vi "UHR-Fleezers Control (host) - 10.8.vi"() -> ()   [LabVIEW 2013] (continued)
          tunnel: [w3020] -> w2914 mode=indexing
          workers-P: _ -> [_]
          n1651 = Reverse 1D Array(array=w3021) -> (reversed array=w3020:dbl[])
        }
        n1652 = for {
          tunnel: w2989 -> [w3029] mode=indexing
          tunnel: [w3028] -> w2988 mode=indexing
          workers-P: _ -> [_]
          n1653 = Reverse 1D Array(array=w3029) -> (reversed array=w3028:dbl[])
        }
        n1654 = for {
          tunnel: w2978 -> [w3025] mode=indexing
          tunnel: [w3024] -> w2977 mode=indexing
          workers-P: _ -> [_]
          n1655 = Reverse 1D Array(array=w3025) -> (reversed array=w3024:dbl[])
        }
        n1656 = Index Array(array=w2990, index (row)=0) -> (element=→"Waveform Graph":dbl[])  [unwired: 1 in]
        n1657 = Add(x=w2984, y=w2983) -> (x+y=w2982:dbl[][])
        n1658 = Add(x=w2970, y=w2969) -> (x+y=w2968:dbl[][])
        n1659 = Add(x=w2914, y=w2913) -> (x+y=w2898:dbl[][])
        n1660 = Add(x=w2988, y=w2987) -> (x+y=w2962:dbl[][])
        n1661 = Add(x=w2977, y=w2976) -> (x+y=w2975:dbl[][])
        n1662 = Divide(x=w2968, y=2) -> (x/y=w2966:dbl[][])
        n1663 = Divide(x=w2982, y=2) -> (x/y=w2927:dbl[][])
        n1664 = Divide(x=w2975, y=2) -> (x/y=w2929:dbl[][])
        n1665 = To Single Precision Float(number=w2962) -> (single precision float=w2961:sgl[][])
        n1666 = Transpose 2D Array(2D array=w2966) -> (transposed array=→"Data map":dbl[][])
        n1667 = To Single Precision Float(number=w2898) -> (single precision float=w2902:sgl[][])
        n1668 = To Single Precision Float(number=w2927) -> (single precision float=w2933:sgl[][])
        n1669 = To Single Precision Float(number=w2929) -> (single precision float=w2930:sgl[][])
        n1670 = call "IMAQ ArrayToImage"("Image Pixels (Float)"=w2961, "Image"=w2895) -> ("Image Out"=w2964:T2)  [unwired: 8 in, 1 out]
        n1671 = call "IMAQ ArrayToImage"("Image Pixels (Float)"=w2902, "Image"=w2894) -> ("Image Out"=w2904:T2)  [unwired: 8 in, 1 out]
        n1672 = call "IMAQ ArrayToImage"("Image Pixels (Float)"=w2933, "Image"=w2893) -> ("Image Out"=w2935:T2)  [unwired: 8 in, 1 out]
        n1673 = call "IMAQ ArrayToImage"("Image Pixels (Float)"=w2930, "Image"=w2892) -> ("Image Out"=w2932:T2)  [unwired: 8 in, 1 out]
        n1674 = call "IMAQ Symmetry"("Type of Symmetry"=w2963, "Image Src"=w2964) -> ("Image Dst Out"=w2959:T2)  [unwired: 3 in, 1 out]
        n1675 = call "IMAQ Symmetry"("Type of Symmetry"=w2903, "Image Src"=w2904) -> ("Image Dst Out"=w2900:T2)  [unwired: 3 in, 1 out]
        n1676 = call "IMAQ Symmetry"("Type of Symmetry"=w2934, "Image Src"=w2935) -> ("Image Dst Out"=→"Detection Laser X":T2)  [unwired: 3 in, 1 out]
        n1677 = call "IMAQ Symmetry"("Type of Symmetry"=w2931, "Image Src"=w2932) -> ("Image Dst Out"=→"Detection Laser Y":T2)  [unwired: 3 in, 1 out]
        n1678 = call "IMAQ Set Simple Calibration"("Calibration Axis Info"=T39 {"Origin Pixel"={"X"=0.0, "Y"=0.0}, "Angle Relative to Horizontal (deg)"=0.0, "Axis Reference"=0}, "Grid Descriptor"=T40 {"X Step"=0.3, "Y Step"=0.3, "Unit"=enum."Undefined"}, "Image"=w2959) -> ("Calibrated Image"=→"APD 1":T2)  [unwired: 7 in, 1 out]
        n1679 = call "IMAQ Set Simple Calibration"("Calibration Axis Info"=T39 {"Origin Pixel"={"X"=0.0, "Y"=0.0}, "Angle Relative to Horizontal (deg)"=0.0, "Axis Reference"=0}, "Grid Descriptor"=T40 {"X Step"=0.3, "Y Step"=0.3, "Unit"=enum."Undefined"}, "Image"=w2900) -> ("Calibrated Image"=→"APD 2":T2)  [unwired: 7 in, 1 out]
      }
    }
    n1680 = Subtract(x=w1995, y="APD 2 Offset") -> (x-y=w1992:waveform(dbl))
    n1681 = Subtract(x=w1997, y="APD 1 Offset") -> (x-y=w1993:waveform(dbl))
    n1682 = Index Array(array=w2012, index=3) -> (element=w2081:waveform(dbl))
    n1683 = Index Array(array=w2012, index=6) -> (element=w2078:waveform(dbl))
    n1684 = Build Array(w1993, w1992) -> (→"APD Chart":waveform(dbl)[])
    n1685 = Array Size(array=w2070) -> (size(s)=w2125:i32)
    n1686 = call <vilib>:"Std Deviation and Variance.vi"("X"=w2005) -> ("standard deviation"=w2004:dbl)  [unwired: 1 in, 2 out]
    n1687 = Add Array Elements(numeric array=w2005) -> (sum=w2007:u32)
    n1688 = Add Array Elements(numeric array=w2070) -> (sum=w2135:u32)
    n1689 = call <vilib>:"Std Deviation and Variance.vi"("X"=w2070) -> ("standard deviation"=w2069:dbl)  [unwired: 1 in, 2 out]
    n1690 = Divide(x="T1 offset_x (mV)", y=1000.0) -> (x/y=w2082:dbl)
    n1691 = Divide(x=w2004, y=w2003) -> (x/y=w2000:dbl)
    "Rate sigma (Hz) 2" <- w2000
    n1692 = Multiply(x=w2003, y=w2125) -> (x*y=w2006:dbl)
    "Int. Time (s)" <- w2006
    n1693 = Divide(x=w2007, y=w2006) -> (x/y=w2001:dbl)
    "APD 2 Rate (Hz)" <- w2001
    n1694 = Divide(x=w2135, y=w2006) -> (x/y=w2067:dbl)
    "APD 1 Rate (Hz)" <- w2067
    n1695 = Divide(x=w2069, y=w2003) -> (x/y=w2068:dbl)
    "Rate sigma (Hz)" <- w2068
    n1696 = Divide(x=w2000, y=w2001) -> (x/y=→"Sigma/Mean 2":dbl)
    n1697 = Divide(x=w2068, y=w2067) -> (x/y=→"Sigma/Mean":dbl)
    n1698 = Divide(x="T2 offset_x (mV)", y=1000.0) -> (x/y=w2080:dbl)
    n1699 = case shown="1" "Calibration" {
      tunnel: "T1 alpha_x (nm/V)" -> [_ w2858 w2879]
      tunnel: "T1 kappa_x (pN/nm)" -> [_ _ w2869]
      tunnel: "T2 alpha_x (nm/V)" -> [_ w2857 w2877]
      tunnel: "T2 kappa_x (pN/nm)" -> [_ _ w2870]
      tunnel: w2081 -> [w2840 w2855 w2875]
      tunnel: w2078 -> [w2839 w2853 w2873]
      tunnel: [w2840 w2852 w2872] -> w2111
      tunnel: [w2839 w2851 w2871] -> w2110
      tunnel: ["T1 X (V)" ("Label.Text") "T1 X (nm)" ("Label.Text") "T1 X (pN)" ("Label.Text")] -> w2099
      tunnel: ["T2 X (V)" ("Label.Text") "T2 X (nm)" ("Label.Text") "T2 X (pN)" ("Label.Text")] -> w2098
      tunnel: ["Position (V)" ("Label.Text") "Position (nm)" ("Label.Text") "Force (pN)" ("Label.Text")] -> w2100
      tunnel: w2080 -> [_ w2843 w2862]
      tunnel: w2082 -> [_ w2846 w2864]
      tunnel: ["Mean (V)" ("Label.Text") "Mean (nm)" ("Label.Text") "Mean (pN)" ("Label.Text")] -> w2095
      tunnel: ["Difference (V)" ("Label.Text") "Difference (nm)" ("Label.Text") "Difference (pN)" ("Label.Text")] -> w2020
      frame 0, Default {
      }
      frame 1 {
        # "position"
        n1700 = Unbundle By Name(w2855) -> ("Y"=w2859:dbl[])
        n1701 = Unbundle By Name(w2853) -> ("Y"=w2844:dbl[])
        n1702 = Subtract(x=w2859, y=w2846) -> (x-y=w2847:dbl[])
        n1703 = Subtract(x=w2844, y=w2843) -> (x-y=w2845:dbl[])
        n1704 = Multiply(x=w2845, y=w2857) -> (x*y=w2854:dbl[])
        n1705 = Multiply(x=w2858, y=w2847) -> (x*y=w2856:dbl[])
        n1706 = Bundle By Name(cluster=w2853, "Y"=w2854) -> (w2851:waveform(dbl))
        n1707 = Bundle By Name(cluster=w2855, "Y"=w2856) -> (w2852:waveform(dbl))
      }
      frame 2 {
        # "force"
        n1708 = Unbundle By Name(w2875) -> ("Y"=w2880:dbl[])
        n1709 = Unbundle By Name(w2873) -> ("Y"=w2878:dbl[])
        n1710 = Subtract(x=w2878, y=w2862) -> (x-y=w2863:dbl[])
        n1711 = Subtract(x=w2880, y=w2864) -> (x-y=w2865:dbl[])
        n1712 = Compound Arithmetic op=MULTIPLY(w2863, w2877, w2870) -> (w2874:dbl[])
        n1713 = Compound Arithmetic op=MULTIPLY(w2869, w2879, w2865) -> (w2876:dbl[])
        n1714 = Bundle By Name(cluster=w2873, "Y"=w2874) -> (w2871:waveform(dbl))
        n1715 = Bundle By Name(cluster=w2875, "Y"=w2876) -> (w2872:waveform(dbl))
      }
    }
    n1716 = feedback-in #17("Calibration") -> ()
    n1717 = feedback #17(u16 1 ("Calibration")) -> (w2102:u16)
    n1718 = Not Equal?(x=w2102, y="Calibration") -> (x != y?=w2058:bool)
    n1719 = Unbundle By Name(w2081) -> ("Y"=w2084:dbl[])
    n1720 = Unbundle By Name(w2078) -> ("Y"=w2087:dbl[])
    n1721 = Subtract(x=w2084, y=w2082) -> (x-y=w2085:dbl[])
    n1722 = Subtract(x=w2087, y=w2080) -> (x-y=w2086:dbl[])
    n1723 = disable-structure shown="Enabled" {
      disable-tunnel: [-1.0 ("y") 1.0] -> w2088
      frame Disabled {
      }
      frame Enabled {
      }
    }
    n1724 = Multiply(x=w2086, y="T2 alpha_x (nm/V)") -> (x*y=w2077:dbl[])
    n1725 = Multiply(x="T1 alpha_x (nm/V)", y=w2085) -> (x*y=w2076:dbl[])
    n1726 = Multiply(x=w2110, y=w2088) -> (x*y=w2089:waveform(dbl))
    n1727 = case shown="True" "Read Lateness and Rel Phase" {
      tunnel: w1912 -> [w2415 w2437]
      tunnel: w1911 -> [w2416 w2436]
      tunnel: [w2415 w2435] -> w2073
      tunnel: [w2416 w2434] -> w2072
      frame False {
      }
      frame True {
        n1728 = xnode "Read/Write Control"("FPGA VI Reference In"=w2437, "error in"=w2436) -> ("FPGA VI Reference Out"=w2435:T19, "error out"=w2434:errorcluster, "GI Relative phase"=→"GI relative phase":i16, "Relative phase"=→"Relative phase (AI1)":i16, "AI Late Counter"=→"Late Counter (AI1)":u16, "GI Late Counter"=→"GI Late Counter":u16, "MCL Late Counter"=→"MCL Late Counter":u16, "MCL Relative Phase"=→"Relative Phase (MCL)":i16, "APD Acq Relative Phase"=→"APD Acq Relative Phase":i16, "APD 1 Gate Relative Phase"=→"APD 1 Gate Relative Phase":i16, "APD 2 Gate Relative Phase"=→"APD 2 Gate Relative Phase":i16, "APD Acq Late Counter"=→"APD Acq Late Counter":u16, "APD 1 Gate Late Counter"=→"APD 1 Gate Late Counter":u16, "APD 2 Gate Late Counter"=→"APD 2 Gate Late Counter":u16, "Green FB Relative Phase"=→"Relative phase (Green FB)":i16, "GI Relative phase 2"=→"GI relative phase 2":i16, "GI Late Counter 2"=→"GI Late Counter 2":u16, "Trap Pos FIFO Timeout"=→"Trap Pos FIFO Timeout":u16, "Trap AI FIFO Timeout"=→"Trap AI FIFO Timeout":u16)
      }
    }
    n1729 = Subtract(x=w2077, y=w2076) -> (x-y=w2075:dbl[])
    n1730 = Unbundle By Name(w2110) -> ("Y"=w2045:dbl[])
    n1731 = Unbundle By Name(w2111) -> ("Y"=w2046:dbl[])
    n1732 = Build Array(w2111, w2089) -> (→"Force":waveform(dbl)[])
    n1733 = Subtract(x=w2075, y="Offset (nm)") -> (x-y=w2043:dbl[])
    n1734 = call-poly <vilib>:"Mean.vi"("X"=w2045) -> ("mean"=w2024:dbl)  [unwired: 1 out]
    "T2 X" <- w2024
    n1735 = Absolute Value(x=w2046) -> (abs(x)=w2047:dbl[])
    n1736 = Absolute Value(x=w2045) -> (abs(x)=w2048:dbl[])
    n1737 = call-poly <vilib>:"Mean.vi"("X"=w2046) -> ("mean"=w2025:dbl)  [unwired: 1 out]
    "T1 X" <- w2025
    n1738 = Add(x=w2047, y=w2048) -> (x+y=w2049:dbl[])
    n1739 = Bundle By Name(cluster=w2081, "Y"=w2043) -> (w2011:waveform(dbl))
    "Bead Separation" <- w2011
    n1740 = Divide(x=w2049, y=2.0) -> (x/y=→"Vec Mean of T1 T2":dbl[])
    n1741 = case shown="True" w2058 {
      tunnel: w2100 -> [_ w2833]
      tunnel: w2099 -> [_ w2832]
      tunnel: w2098 -> [_ w2831]
      tunnel: w2095 -> [_ w2830]
      tunnel: w2020 -> [_ w2829]
      frame False {
      }
      frame True {
        n1742 = property on="Force" class="WFChart (strict)"("YScale.NameLbl.Text"=w2833) -> ()  [unwired: 2 in, 2 out]
        n1743 = property on="T2 X" class="DigNum (strict)"("Caption.Text"=w2831) -> ()  [unwired: 2 in, 2 out]
        n1744 = property on="T1 X" class="DigNum (strict)"("Caption.Text"=w2832) -> ()  [unwired: 2 in, 2 out]
        n1745 = property on="Mean" class="DigNum (strict)"("Caption.Text"=w2830) -> ()  [unwired: 2 in, 2 out]
        n1746 = property on="Difference" class="DigNum (strict)"("Caption.Text"=w2829) -> ()  [unwired: 2 in, 2 out]
      }
    }
    n1747 = local read "Tether"() -> (w2052:bool)
    n1748 = Absolute Value(x=w2025) -> (abs(x)=w2022:dbl)
    n1749 = Absolute Value(x=w2024) -> (abs(x)=w2021:dbl)
    n1750 = Add(x=w2022, y=w2021) -> (x+y=w2097:dbl)
    n1751 = Subtract(x=w2022, y=w2021) -> (x-y=→"Difference":dbl)
    n1752 = feedback #18(w2043) -> (w2042:dbl[])
    n1753 = Divide(x=w2097, y=2.0) -> (x/y=w2051:dbl)
    "Mean" <- w2051
    n1754 = case shown="True" w2052 {
      tunnel: w2051 -> [_ w2374]
      frame False {
      }
      frame True {
        n1755 = Greater?(x="Lost Tether Alarm Threshold (pN)", y=w2374) -> (0:w2372:bool)
        n1756 = case shown="True" w2372 {
          frame False {
          }
          frame True {
            n1757 = flat-sequence {
              frame #0 {
                # "stop only if saving"
                n1758 = local read "Saving..."() -> (w2387:bool)
                n1759 = And(x=w2387, y="TA Cancel Save?") -> (x .and. y?=w2386:bool)
                n1760 = local write "Stop Saving"(w2386) -> ()
              }
              frame #1 {
                n1761 = case shown="True" "TA Green Off?" {
                  frame False {
                  }
                  frame True {
                    w2390 = FALSE ("Fl. Triggered...")
                    n1762 = local write "Fl. Triggered..."(w2390) -> ()
                    n1763 = property on="Green Laser ON/Interlacing" class="Bool (strict)"("Val(Sgnl)"=w2390) -> ()  [unwired: 2 in, 2 out]
                  }
                }
              }
            }
            n1764 = local read "Time tether formed"() -> (w2381:timestamp)
            n1765 = Get Date/Time In Seconds() -> (seconds since 1Jan1904=w2382:timestamp)
            n1766 = Subtract(x=w2382, y=w2381) -> (x-y=w2380:dbl)
            n1767 = Number To Decimal String(number=w2380) -> (decimal integer string=w2377:string)  [unwired: 1 out]
            n1768 = local read "Messages"() -> (w2384:string)
            n1769 = call <vilib>:"Beep.vi"() -> ()  [unwired: 3 in, 9 out]
            n1770 = Concatenate Strings("Lost tether (" ("Message to add"), w2377, " s)." ("string")) -> (w2379:string)
            n1771 = local write "Tether"(FALSE ("Tether")) -> ()
            n1772 = call "Update messages.vi"("Message to add"=w2379, "Old message string"=w2384) -> ("New message string"=w2383:string)
            n1773 = local write "Messages"(w2383) -> ()
            n1774 = property on="Trap Pos. FB ON" class="Bool (strict)"("Val(Sgnl)"=FALSE ("Value (Signaling)")) -> ()  [unwired: 2 in, 2 out]
          }
        }
      }
    }
    n1775 = Build Array (concatenate)(w2043, w2042) -> (w2041:dbl[])
    n1776 = Split 1D Array(array=w2041, index=w1923) -> (first subarray=w2037:dbl[])  [unwired: 1 out]
    n1777 = feedback-in #18(w2037) -> ()
    n1778 = call-poly <vilib>:"Mean.vi"("X"=w2037) -> ("mean"=w2036:dbl)  [unwired: 1 out]
    "Bead Mean (nm)" <- w2036
    n1779 = Subtract(x=w2037, y=w2036) -> (x-y=w2035:dbl[])
    n1780 = Square(x=w2035) -> (x^2=w2034:dbl[])
    n1781 = call-poly <vilib>:"Mean.vi"("X"=w2034) -> ("mean"=w2033:dbl)  [unwired: 1 out]
    n1782 = Square Root(x=w2033) -> (sqrt(x)=w2032:dbl)
    n1783 = Multiply(x=10.0, y=w2032) -> (x*y=→"RMS (Ang)":dbl)
    n1784 = xnode "Read/Write Control"("FPGA VI Reference In"=w2073, "error in"=w2072) -> ("FPGA VI Reference Out"=w2191:T19, "error out"=w2185:errorcluster, "AI2 Y Sum Set 1"=w2181:i16, "AI2 Y Sum Set 2"=w2180:i16, "AI1 X Set 1"=w1957:fxp<+/-,16,1>, "AI1 X Set 2"=w1956:fxp<+/-,16,1>, "Trap Pos FB Int Signal"=→"Trap Pos FB Int Signal":fxp<+/-,24,9>, "Trap Pos FB Int-Norm Signal"=→"Trap Pos FB Int-Norm Signal":fxp<+/-,16,1>, "Trap Pos FB Action"=w1950:i64, "Scanning"=→"AOD Scanning":bool, "Scan I"=→"AOD Scan I":u64, "Scanning MCL"=w2183:bool, "Scan I (MCL)"=→"MCL Scan I":u64, "Green FB Signals"=w2120:T44)  [unwired: 1 out]
    "MCL Scanning" <- w2183
    "Trap Pos FB Action" <- w1950
    n1785 = local read "AI2 (V)"() -> (w2182:cluster{"Set 1":dbl, "Set 2":dbl})
    n1786 = Bundle By Name(cluster=w2182, "Set 1"=w2181, "Set 2"=w2180) -> (w2178:cluster{"Set 1":dbl, "Set 2":dbl})
    n1787 = Divide(x=w1950, y=327.67) -> (x/y=→"Action (%)":dbl)
    n1788 = local read "Trap X (AI1)"() -> (w1970:T10)
    n1789 = Divide(x=w2178, y=3276.7) -> (x/y=w2177:cluster{"Set 1":dbl, "Set 2":dbl})
    n1790 = local write "AI2 (V)"(w2177) -> ()
    n1791 = Bundle(cluster=w1970, "Trap 1"=w1957, "Trap 2"=w1956) -> (→"Trap X (AI1)":T10)
    n1792 = Divide(x=w2120, y=3276.7) -> (x/y=w2116:T51)
    n1793 = Unbundle By Name(w2116) -> ("Green FB Ch 0"=w2119:dbl, "Green FB Ch 1"=w2118:dbl, "Green FB Ch 2"=w2117:dbl)
    n1794 = Divide(x=w2119, y=w2117) -> (x/y=w2115:dbl)
    n1795 = Divide(x=w2118, y=w2117) -> (x/y=w2114:dbl)
    n1796 = flat-sequence "To save data" {
      tunnel: [w4117] -> w2202
      tunnel: [w4118] -> w2201
      tunnel: w2151 -> [w4111]
      tunnel: w2039 -> [w4115]
      tunnel: ["Save Calibration"] -> w2174
      tunnel: w2171 -> [w4114]
      tunnel: [w4107] -> w2170
      tunnel: [w4104] -> w2169
      tunnel: [w4101] -> w2168
      tunnel: w2150 -> [w4103]
      tunnel: w2056 -> [w4097]
      tunnel: [w4097] -> w2055
      tunnel: ["Start Saving"] -> w2013
      tunnel: [w4091] -> w1939
      tunnel: [w4090] -> w1938
      tunnel: w2202 -> [w4352]
      tunnel: w2201 -> [w4351]
      tunnel: w1940 -> [w4350]
      tunnel: w2174 -> [w4349]
      tunnel: w2170 -> [w4347]
      tunnel: w2169 -> [w4346]
      tunnel: w2168 -> [w4345]
      tunnel: w2026 -> [w4344]
      tunnel: w2065 -> [w4343]
      tunnel: w2055 -> [w4342]
      tunnel: w2013 -> [w4341]
      tunnel: w2011 -> [w4340]
      tunnel: w1987 -> [w4339]
      tunnel: w1939 -> [w4338]
      tunnel: w1938 -> [w4337]
      tunnel: w1937 -> [w4336]
      frame #0 {
        n1797 = Or(x="Save N Sets", y="Start Saving") -> (x .or. y?=w4098:bool)
        n1798 = To Double Precision Float(number=w4114) -> (double precision float=w4108:dbl)
        n1799 = Build Array(w4098, "Save Calibration", w4111, w4103) -> (w4113:bool[])
        n1800 = Compound Arithmetic op=OR("Save Calibration", w4111, w4098, w4103) -> (w4116:bool)
        n1801 = Boolean Array To Number(Boolean array=w4113) -> (number=w4110:u32)
        n1802 = feedback #19(FALSE ("Save APD Data\nwith Trap Data")) -> (w4092:bool)
        n1803 = feedback #20(refnum<k0> refnum) -> (w4119:refnum<file>)
        n1804 = feedback #21(refnum<k0> refnum) -> (w4094:refnum<file>)
        n1805 = feedback #22(FALSE ("Save APD Data\nwith Trap Data")) -> (w4102:bool)
        n1806 = feedback #23(refnum<k0> refnum) -> (w4105:refnum<file>)
        n1807 = feedback #24(0) -> (w4121:i32)
        n1808 = feedback #25() -> (w4109:u32)  [unwired: 1 out]
        n1809 = case shown="True" w4116 {
          tunnel: [w4128 1] -> w4117
          tunnel: w4121 -> [w4130 _]
          tunnel: [w4129 w4148] -> w4118
          tunnel: w4119 -> [w4129 _]
          tunnel: w4115 -> [_ w4168]
          tunnel: w4108 -> [_ w4166]
          tunnel: w4110 -> [_ w4169]
          tunnel: [w4127 w4147] -> w4107
          tunnel: w4109 -> [w4127 _]
          tunnel: [w4126 w4145] -> w4104
          tunnel: w4105 -> [w4126 _]
          tunnel: [w4125 w4144] -> w4101
          tunnel: w4102 -> [w4125 _]
          tunnel: "Start Saving" -> [_ w4142]
          tunnel: w4097 -> [_ w4141]
          tunnel: [w4124 w4132] -> w4090
          tunnel: w4094 -> [w4124 _]
          tunnel: [w4123 w4131] -> w4091
          tunnel: w4092 -> [w4123 _]
          frame False {
            n1810 = Increment(x=w4130) -> (x+1=w4128:i32)
          }
          frame True {
            w4138 = FALSE ("Start Saving")
            w4143 = 9.0  # File Version
            w4151 = FALSE ("prepend array or string size? (T)")
            w4149 = T31."big-endian, network order" ("byte order (0:big-endian, network order)")
            # "write file headers"
            n1811 = local read "BD 1 Frequency 1 (MHz)"() -> (w4165:dbl)
            n1812 = local read "BD 2 Frequency 1 (MHz)"() -> (w4164:dbl)
            n1813 = local read "BD 1 Frequency 2 (MHz)"() -> (w4163:dbl)
            n1814 = local read "BD 2 Frequency 2 (MHz)"() -> (w4162:dbl)
            n1815 = local read "BD 1 Frequency 3 (MHz)"() -> (w4161:dbl)
            n1816 = local read "BD 2 Frequency 3 (MHz)"() -> (w4160:dbl)
            n1817 = Array Size(array=w4141) -> (size(s)=w4140:i32)
            n1818 = To Double Precision Float(number=w4140) -> (double precision float=w4139:dbl)
            n1819 = local write "Save Calibration"(w4138) -> ()
            n1820 = local write "Start Saving"(w4138) -> ()
            n1821 = Build Array("Save APD Data\nwith Trap Data", "Save Trap Pos. Data") -> (w4135:bool[])
            n1822 = Boolean Array To Number(Boolean array=w4135) -> (number=w4134:u32)
            n1823 = Build Array(w4165, w4164, w4163, w4162, w4161, w4160) -> (w4159:dbl[])
            n1824 = case shown="4" w4169 {
              tunnel: w4168 -> [w4240 w4260 w4276 w4314]
              tunnel: w4139 -> [w4245 w4267 w4296 w4333]
              tunnel: w4166 -> [w4244 w4266 w4295 w4332]
              tunnel: [w4241 w4262 w4287 w4324] -> w4157
              tunnel: [w4232 "Cal sets to save" w4277 w4315] -> w4147
              tunnel: w4159 -> [w4242 w4263 w4289 w4326]
              tunnel: "Save APD Data\nwith Trap Data" -> [w4239 _ w4273 w4312]
              tunnel: [w4239 w4254 w4273 w4312] -> w4144
              tunnel: w4143 -> [w4235 w4255 w4271 w4310]
              tunnel: w4142 -> [w4234 _ _ _]
              tunnel: [w4225 w4254 w4270 w4300] -> w4131
              tunnel: "Save Trap Pos. Data" -> [w4225 _ w4270 w4300]
              tunnel: w4134 -> [w4224 _ w4269 w4299]
              frame 1, Default {
                # "timeseries"
                n1825 = case shown="True" "Profile" {
                  tunnel: [w4248 w4251] -> w4229
                  tunnel: [w4248 w4250] -> w4228
                  tunnel: [w4248 w4249] -> w4227
                  tunnel: [w4248 w4253] -> w4226
                  frame False {
                    w4248 = 0.0 ("f")
                  }
                  frame True {
                    n1826 = local read "Current Position"() -> (w4252:dbl[])
                    n1827 = local read "Y change (mm)"() -> (w4253:dbl)
                    n1828 = call "subVI_explode3array.vi"("Array"=w4252) -> ("x"=w4251:dbl, "y"=w4250:dbl, "z"=w4249:dbl)  [unwired: 12 in]
                  }
                }
                n1829 = local read "Save ave N"() -> (w4247:dbl)
                n1830 = Multiply(x=w4247, y=w4240) -> (x*y=w4246:dbl)
                n1831 = To Double Precision Float(number=w4224) -> (double precision float=w4238:dbl)
                n1832 = Build Array(w4235, w4240, w4246, w4245, w4244, 0.0 ("f")) -> (w4243:dbl[])
                n1833 = Build Array(w4238, w4229, w4228, w4227, w4226) -> (w4236:dbl[])
                n1834 = Select(t=u32 4000000000, s=w4234, f="N sets to save") -> (s? t:f=w4232:u32)
                n1835 = Build Array (concatenate)(w4243, w4242, w4236) -> (w4241:dbl[])
              }
              frame 2 {
                w4257 = 0.0 ("f")
                w4254 = FALSE ("Save APD Data\nwith Trap Data")
                # "calibration"
                n1836 = Boolean To (0,1)(Boolean=w4254) -> (0, 1=w4259:i16)
                n1837 = To Double Precision Float(number=w4259) -> (double precision float=w4258:dbl)
                n1838 = Build Array(w4258, w4257, w4257, w4257, w4257) -> (w4256:dbl[])
                n1839 = Build Array(w4255, w4260, w4260, w4267, w4266, 1.0 ("t")) -> (w4264:dbl[])
                n1840 = Build Array (concatenate)(w4264, w4263, w4256) -> (w4262:dbl[])
                "Calibrating Trap..." <- TRUE ("Calibrating...")
              }
              frame 4 {
                w4274 = 0.0 ("f")
                # "write file header for a trap \nraster scan"
                # "scan dir (x/y = 0/1)"
                # "cycles/step"
                # "n scans (f/b)"
                # "steps"
                # "freq. range"
                # "AOD raster scan"
                n1841 = local read "Number of F/B Scans (AOD)"() -> (w4281:u16)
                n1842 = local read "Cycles/step (AOD)"() -> (w4283:u64)
                n1843 = local read "Scan Range (MHz)"() -> (w4286:dbl)
                n1844 = local read "Scan steps (AOD)"() -> (w4285:u64)
                n1845 = local read "Scan BD"() -> (w4293:bool)
                n1846 = local read "Save ave N"() -> (w4298:dbl)
                n1847 = Boolean To (0,1)(Boolean=w4293) -> (0, 1=w4292:i16)
                n1848 = To Double Precision Float(number=w4281) -> (double precision float=w4280:dbl)
                n1849 = To Double Precision Float(number=w4285) -> (double precision float=w4284:dbl)
                n1850 = To Double Precision Float(number=w4283) -> (double precision float=w4282:dbl)
                n1851 = To Double Precision Float(number=w4292) -> (double precision float=w4291:dbl)
                n1852 = Multiply(x=w4298, y=w4276) -> (x*y=w4297:dbl)
                n1853 = To Double Precision Float(number=w4269) -> (double precision float=w4275:dbl)
                n1854 = Build Array(w4275, w4274, w4274, w4274, w4274) -> (w4272:dbl[])
                n1855 = local read "N sets should be saved"() -> (w4278:dbl)
                n1856 = Build Array(w4291, w4286, w4284, w4282, w4280) -> (w4288:dbl[])
                n1857 = Build Array(w4271, w4276, w4297, w4296, w4295, 2.0 ("t")) -> (w4290:dbl[])
                n1858 = Round Toward +Infinity(x=w4278) -> (ceil(x): smallest int >= x=w4279:dbl)
                n1859 = Build Array (concatenate)(w4290, w4289, w4272, w4288) -> (w4287:dbl[])
                n1860 = To Unsigned Long Integer(number=w4279) -> (unsigned 32bit integer=w4277:u32)
              }
              frame 8 {
                w4307 = 0.0 ("f")
                # "MCL raster scan"
                n1861 = local read "Number of scans (MCL)"() -> (w4302:u64)
                n1862 = local read "Scan lines (y)"() -> (w4301:u64)
                n1863 = local read "2D or 1D Scan"() -> (w4304:bool)
                n1864 = local read "Scan Range (V)\n(of steps)"() -> (w4323:dbl)
                n1865 = local read "Fast Scan Dir"() -> (w4330:bool)
                n1866 = local read "Cycles/step (MCL)"() -> (w4320:u64)
                n1867 = local read "Scan steps (MCL)"() -> (w4322:u64)
                n1868 = Select(t=w4301, s=w4304, f=w4302) -> (s? t:f=w4303:u64)
                n1869 = Boolean To (0,1)(Boolean=w4304) -> (0, 1=w4306:i16)
                n1870 = local read "Save ave N"() -> (w4335:dbl)
                n1871 = local read "Initial X"() -> (w4309:dbl)
                n1872 = local read "Initial Y"() -> (w4308:dbl)
                n1873 = To Double Precision Float(number=w4306) -> (double precision float=w4305:dbl)
                n1874 = Boolean To (0,1)(Boolean=w4330) -> (0, 1=w4329:i16)
                n1875 = To Double Precision Float(number=w4303) -> (double precision float=w4318:dbl)
                n1876 = To Double Precision Float(number=w4322) -> (double precision float=w4321:dbl)
                n1877 = To Double Precision Float(number=w4320) -> (double precision float=w4319:dbl)
                n1878 = To Double Precision Float(number=w4329) -> (double precision float=w4328:dbl)
                n1879 = Multiply(x=w4335, y=w4314) -> (x*y=w4334:dbl)
                n1880 = To Double Precision Float(number=w4299) -> (double precision float=w4313:dbl)
                n1881 = local read "N sets should be saved (MCL)"() -> (w4316:dbl)
                n1882 = Build Array(w4313, w4305, w4307, w4307, w4307) -> (w4311:dbl[])
                n1883 = Build Array(w4328, w4323, w4321, w4319, w4318, w4309, w4308) -> (w4325:dbl[])
                n1884 = Build Array(w4310, w4314, w4334, w4333, w4332, 3.0 ("t")) -> (w4327:dbl[])
                n1885 = Round Toward +Infinity(x=w4316) -> (ceil(x): smallest int >= x=w4317:dbl)
                n1886 = Build Array (concatenate)(w4327, w4326, w4311, w4325) -> (w4324:dbl[])
                n1887 = To Unsigned Long Integer(number=w4317) -> (unsigned 32bit integer=w4315:u32)
              }
            }
            n1888 = local read "Index"() -> (w4174:dbl)
            n1889 = call "Create new save file.vi"("Insert"="", "Ext"=".dat", "Index In"=w4174) -> ("Path Out"=w4133:path, "Index Out"=w4146:dbl)
            n1890 = local write "Save file name"(w4133) -> ()
            n1891 = local write "Index"(w4146) -> ()
            n1892 = local write "Save index"(w4146) -> ()
            n1893 = Array Size(array=w4157) -> (size(s)=w4158:i32)
            n1894 = Open/Create/Replace File(file path (use dialog)=w4133, operation (0:open)=T23."create", access (0:read/write)=enum16{"read/write", "read-only", "write-only"}."write-only") -> (refnum out=w4171:refnum<file>)  [unwired: 1 in, 4 out]
            n1895 = local write "Saving..."(TRUE ("Saving...")) -> ()
            n1896 = To Double Precision Float(number=w4158) -> (double precision float=w4156:dbl)
            n1897 = String Length(string="Comment (data description)") -> (length=w4154:i32)
            n1898 = To Double Precision Float(number=w4154) -> (double precision float=w4153:dbl)
            n1899 = Deny Access(7:w4171) -> (3:w4170:refnum<file>)  [unwired: 1 in, 2 out]
            n1900 = Build Array (concatenate)(w4156, w4157, w4153) -> (w4155:dbl[])
            n1901 = case "If fluorescence data to be saved" shown="True" w4144 {
              tunnel: w4133 -> [_ w4223]
              tunnel: [refnum<k0> refnum w4203] -> w4145
              frame False {
              }
              frame True {
                w4202 = 0.0
                n1902 = local read "APD Integration Time (s)"() -> (w4208:dbl)
                n1903 = local read "N APD Samp/step"() -> (w4201:dbl)
                n1904 = Path To String(path=w4223) -> (string=w4222:string)
                n1905 = String Length(string=w4222) -> (length=w4221:i32)
                n1906 = Subtract(x=w4221, y=4) -> (x-y=w4219:i32)
                n1907 = String Subset(string=w4222, length (rest)=w4219) -> (substring=w4218:string)  [unwired: 1 out]
                n1908 = Build Array(w4208, w4201, w4202, w4202, w4202, w4202, w4202, w4202) -> (w4205:dbl[])
                n1909 = Concatenate Strings(w4218, "_fl.dat" ("string")) -> (w4216:string)
                n1910 = Array Size(array=w4205) -> (size(s)=w4207:i32)
                n1911 = String To Path(string=w4216) -> (path=w4212:path)
                n1912 = Open/Create/Replace File(file path (use dialog)=w4212, operation (0:open)=T23."create", access (0:read/write)=enum16{"read/write", "read-only", "write-only"}."write-only") -> (refnum out=w4213:refnum<file>)  [unwired: 1 in, 4 out]
                n1913 = Deny Access(7:w4213) -> (3:w4209:refnum<file>)  [unwired: 1 in, 2 out]
                n1914 = To Double Precision Float(number=w4207) -> (double precision float=w4206:dbl)
                n1915 = Build Array (concatenate)(w4206, w4205) -> (w4204:dbl[])
                n1916 = Write to Binary File(file (use dialog)=w4209, data=w4204, 5:FALSE ("prepend array or string size? (T)"), 9:T31."big-endian, network order" ("byte order (0:big-endian, network order)")) -> (refnum out=w4203:refnum<file>)  [unwired: 1 in, 3 out]
              }
            }
            n1917 = case shown="True" w4131 {
              tunnel: w4133 -> [_ w4185]
              tunnel: [refnum<k0> refnum w4184] -> w4132
              frame False {
              }
              frame True {
                w4180 = 0.0 ("element")
                n1918 = Path To String(path=w4185) -> (string=w4199:string)
                n1919 = Build Array(w4180, w4180, w4180, w4180, w4180, w4180, w4180, w4180) -> (w4181:dbl[])
                n1920 = String Length(string=w4199) -> (length=w4198:i32)
                n1921 = Subtract(x=w4198, y=4) -> (x-y=w4196:i32)
                n1922 = Array Size(array=w4181) -> (size(s)=w4183:i32)
                n1923 = String Subset(string=w4199, length (rest)=w4196) -> (substring=w4195:string)  [unwired: 1 out]
                n1924 = To Double Precision Float(number=w4183) -> (double precision float=w4182:dbl)
                n1925 = Concatenate Strings(w4195, "_pos.dat" ("string")) -> (w4193:string)
                n1926 = Build Array (concatenate)(w4182, w4181) -> (w4179:dbl[])
                n1927 = String To Path(string=w4193) -> (path=w4189:path)
                n1928 = Open/Create/Replace File(file path (use dialog)=w4189, operation (0:open)=T23."create", access (0:read/write)=enum16{"read/write", "read-only", "write-only"}."write-only") -> (refnum out=w4190:refnum<file>)  [unwired: 1 in, 4 out]
                n1929 = Deny Access(7:w4190) -> (3:w4186:refnum<file>)  [unwired: 1 in, 2 out]
                n1930 = Write to Binary File(file (use dialog)=w4186, data=w4179, 5:FALSE ("prepend array or string size? (T)"), 9:T31."big-endian, network order" ("byte order (0:big-endian, network order)")) -> (refnum out=w4184:refnum<file>)  [unwired: 1 in, 3 out]
              }
            }
            n1931 = Write to Binary File(file (use dialog)=w4170, data=w4155, 5:w4151, 9:w4149) -> (refnum out=w4152:refnum<file>)  [unwired: 1 in, 3 out]
            n1932 = Write to Binary File(file (use dialog)=w4152, data="Comment (data description)", 5:w4151, 9:w4149) -> (refnum out=w4148:refnum<file>)  [unwired: 1 in, 3 out]
          }
        }
        n1933 = feedback-in #19(w4091) -> ()
        n1934 = feedback-in #20(w4118) -> ()
        n1935 = feedback-in #21(w4090) -> ()
        n1936 = feedback-in #22(w4101) -> ()
        n1937 = feedback-in #23(w4104) -> ()
        n1938 = feedback-in #24(w4117) -> ()
        n1939 = feedback-in #25(w4107) -> ()
      }
      frame #1 {
        n1940 = local read "Saving..."() -> (w4348:bool)
        n1941 = case shown="True" w4348 {
          tunnel: w4352 -> [_ w4362]
          tunnel: w4351 -> [_ w4376]
          tunnel: w4350 -> [_ w4372]
          tunnel: w4349 -> [_ w4371]
          tunnel: w4347 -> [_ w4370]
          tunnel: w4346 -> [_ w4365]
          tunnel: w4345 -> [_ w4364]
          tunnel: w4344 -> [_ w4363]
          tunnel: w4343 -> [_ w4361]
          tunnel: w4342 -> [_ w4359]
          tunnel: w4341 -> [_ w4358]
          tunnel: w4340 -> [_ w4357]
          tunnel: w4339 -> [_ w4356]
          tunnel: w4338 -> [_ w4355]
          tunnel: w4337 -> [_ w4354]
          tunnel: w4336 -> [_ w4353]
          frame False {
          }
          frame True {
            n1942 = Multiply(x=w4362, y=w4361) -> (x*y=→"Time (s)":dbl)
            n1943 = Less Or Equal?(x=w4362, y=w4370) -> (x <= y?=w4374:bool)
            n1944 = Or(x="Stop Saving", y="Abort save 2") -> (x .or. y?=w4366:bool)
            n1945 = Not(x=w4366) -> (.not. x?=w4375:bool)
            n1946 = And(x=w4374, y=w4375) -> (x .and. y?=w4373:bool)
            n1947 = case shown="False" w4373 {
              tunnel: w4376 -> [w4383 w4451]
              tunnel: [0.0 w4454] -> w4369
              tunnel: w4362 -> [_ w4452]
              tunnel: w4370 -> [_ w4453]
              tunnel: w4372 -> [_ w4448]
              tunnel: w4371 -> [_ _]
              tunnel: w4365 -> [w4381 w4441]
              tunnel: w4364 -> [w4380 w4442]
              tunnel: w4363 -> [_ w4440]
              tunnel: w4359 -> [_ w4439]
              tunnel: w4358 -> [_ w4393]
              tunnel: w4357 -> [_ w4432]
              tunnel: w4356 -> [_ w4410]
              tunnel: w4355 -> [w4378 w4391]
              tunnel: w4354 -> [w4379 w4390]
              tunnel: w4353 -> [_ w4387]
              frame False {
                w4377 = FALSE
                n1948 = Close File(refnum=w4383) -> ()  [unwired: 1 in, 2 out]
                n1949 = case shown="True" w4380 {
                  tunnel: w4381 -> [_ w4385]
                  frame False {
                  }
                  frame True {
                    n1950 = Close File(refnum=w4385) -> ()  [unwired: 1 in, 2 out]
                  }
                }
                n1951 = case shown="True" w4378 {
                  tunnel: w4379 -> [_ w4384]
                  frame False {
                  }
                  frame True {
                    n1952 = Close File(refnum=w4384) -> ()  [unwired: 1 in, 2 out]
                  }
                }
                n1953 = local write "Calibrating Trap..."(w4377) -> ()
                n1954 = call <vilib>:"Beep.vi"() -> ()  [unwired: 3 in, 9 out]
                n1955 = local write "Stop Saving"(w4377) -> ()
                n1956 = property on="Raster Scanning..." class="Bool (strict)"("Val(Sgnl)"=w4377) -> ()  [unwired: 2 in, 2 out]
                "Saving..." <- w4377
              }
              frame True {
                n1957 = local read "Calibrating Trap..."() -> (w4443:bool)
                n1958 = case "Write fl. data" shown="True" w4442 {
                  tunnel: w4441 -> [_ w4477]
                  tunnel: w4440 -> [_ w4476]
                  frame False {
                  }
                  frame True {
                    n1959 = Write to Binary File(file (use dialog)=w4477, data=w4476, 5:FALSE ("prepend array or string size? (T)"), 9:T31."big-endian, network order" ("byte order (0:big-endian, network order)")) -> ()  [unwired: 1 in, 4 out]
                  }
                }
                n1960 = Greater?(x="Save ave N", y=1.0) -> (0:w4446:bool)
                n1961 = Not(x=w4443) -> (.not. x?=w4445:bool)
                n1962 = And(x=w4445, y=w4446) -> (x .and. y?=w4388:bool)
                n1963 = case shown="True" w4388 {
                  tunnel: w4387 -> [w4457 w4468]
                  tunnel: [w4457 w4460] -> w4386
                  tunnel: "Save ave N" -> [_ w4461]
                  frame False {
                  }
                  frame True {
                    w4458 = 2 ("dimension size")
                    n1964 = Array Size(array=w4468) -> (size(s)=w4462:i32)
                    n1965 = Divide(x=w4462, y=w4458) -> (x/y=w4466:dbl)
                    n1966 = Reshape Array(w4468, w4466, w4458) -> (w4467:u64[][])
                    n1967 = Transpose 2D Array(2D array=w4467) -> (transposed array=w4465:u64[][])
                    n1968 = for {
                      tunnel: w4465 -> [w4470] mode=indexing
                      tunnel: [w4469] -> w4459 mode=indexing
                      tunnel: w4461 -> [w4471]
                      workers-P: _ -> [_]
                      n1969 = call "downsample 1D array - U64.vi"("Ave N"=w4471, "Array In"=w4470) -> ("Array Out"=w4469:u64[])  [unwired: 1 in]
                    }
                    n1970 = Transpose 2D Array(2D array=w4459) -> (transposed array=w4464:u64[][])
                    n1971 = Divide(x=w4462, y=w4461) -> (x/y=w4463:dbl)
                    n1972 = Reshape Array(w4464, w4463) -> (w4460:u64[])
                  }
                }
                n1973 = case shown="True" w4388 {
                  tunnel: w4448 -> [w4480 w4492]
                  tunnel: [w4480 w4484] -> w4444
                  tunnel: "Save ave N" -> [_ w4485]
                  tunnel: w4439 -> [_ w4483]
                  frame False {
                    # "don't downsample data for trap calibration"
                  }
                  frame True {
                    n1974 = Array Size(array=w4492) -> (size(s)=w4486:i32)
                    n1975 = Array Size(array=w4483) -> (size(s)=w4482:i32)
                    n1976 = Divide(x=w4486, y=w4482) -> (x/y=w4490:dbl)
                    n1977 = Reshape Array(w4492, w4490, w4482) -> (w4491:i16[][])
                    n1978 = Transpose 2D Array(2D array=w4491) -> (transposed array=w4489:i16[][])
                    n1979 = for {
                      tunnel: w4489 -> [w4495] mode=indexing
                      tunnel: [w4494] -> w4481 mode=indexing
                      tunnel: w4485 -> [w4493]
                      workers-P: _ -> [_]
                      n1980 = call "downsample 1D array - I16.vi"("Ave N"=w4493, "Array In"=w4495) -> ("Array Out"=w4494:i16[])  [unwired: 1 out]
                    }
                    n1981 = Transpose 2D Array(2D array=w4481) -> (transposed array=w4488:i16[][])
                    n1982 = Divide(x=w4486, y=w4485) -> (x/y=w4487:dbl)
                    n1983 = Reshape Array(w4488, w4487) -> (w4484:i16[])
                  }
                }
                n1984 = Index Array(array=w4410, index=1) -> (element=w4413:waveform(dbl))
                n1985 = Index Array(array=w4410, index=0) -> (element=w4415:waveform(dbl))
                n1986 = Unbundle By Name(w4413) -> ("Y"=w4417:dbl[])
                n1987 = Unbundle By Name(w4415) -> ("Y"=w4425:dbl[])
                n1988 = case "Write trap pos. data" shown="True" w4391 {
                  tunnel: w4390 -> [_ w4473]
                  tunnel: w4386 -> [_ w4472]
                  frame False {
                  }
                  frame True {
                    n1989 = Write to Binary File(file (use dialog)=w4473, data=w4472, 5:FALSE ("prepend array or string size? (T)"), 9:T31."big-endian, network order" ("byte order (0:big-endian, network order)")) -> ()  [unwired: 1 in, 4 out]
                  }
                }
                n1990 = Write to Binary File(file (use dialog)=w4451, data=w4444, 5:FALSE ("prepend array or string size? (T)"), 9:T31."big-endian, network order" ("byte order (0:big-endian, network order)")) -> ()  [unwired: 1 in, 4 out]
                n1991 = feedback #26(w4417) -> (w4419:dbl[])
                n1992 = Build Array (concatenate)(w4419, w4417) -> (w4418:dbl[])
                n1993 = Select(t=w4417, s=w4393, f=w4418) -> (s? t:f=w4403:dbl[])
                n1994 = feedback-in #26(w4403) -> ()
                n1995 = feedback #27(w4425) -> (w4438:dbl[])
                n1996 = Build Array (concatenate)(w4438, w4425) -> (w4437:dbl[])
                n1997 = Select(t=w4425, s=w4393, f=w4437) -> (s? t:f=w4412:dbl[])
                n1998 = feedback-in #27(w4412) -> ()
                n1999 = Divide(x=w4452, y=w4453) -> (x/y=w4455:dbl)
                n2000 = Multiply(x=w4455, y=100.0) -> (x*y=w4454:dbl)
                n2001 = Build Array(w4412, w4403) -> (→"Saved APD":dbl[][])
                n2002 = Array Size(array=w4412) -> (size(s)=w4430:i32)
                n2003 = Unbundle By Name(w4432) -> ("Y"=w4436:dbl[])
                n2004 = Subtract(x=w4430, y="N pts to average") -> (x-y=w4406:i32)
                n2005 = Multiply(x="N pts to average", y=u16 2) -> (x*y=w4407:u16)
                n2006 = Subtract(x=w4430, y=w4407) -> (x-y=w4405:i32)
                n2007 = feedback #28(w4436) -> (w4435:dbl[])
                n2008 = Build Array (concatenate)(w4435, w4436) -> (w4434:dbl[])
                n2009 = Select(t=w4436, s=w4393, f=w4434) -> (s? t:f=w4433:dbl[])
                "Trap Delta Graph" <- w4433
                n2010 = feedback-in #28(w4433) -> ()
                n2011 = Array Subset(array=w4412, index=w4406, length="N pts to average") -> (w4429:dbl[])
                n2012 = Array Subset(array=w4412, index=w4405, length="N pts to average") -> (w4428:dbl[])
                n2013 = Array Subset(array=w4403, index=w4406, length="N pts to average") -> (w4409:dbl[])
                n2014 = Array Subset(array=w4403, index=w4405, length="N pts to average") -> (w4408:dbl[])
                n2015 = call-poly <vilib>:"Mean.vi"("X"=w4429) -> ("mean"=w4427:dbl)  [unwired: 1 out]
                n2016 = call-poly <vilib>:"Mean.vi"("X"=w4409) -> ("mean"=w4402:dbl)  [unwired: 1 out]
                n2017 = call-poly <vilib>:"Mean.vi"("X"=w4428) -> ("mean"=w4426:dbl)  [unwired: 1 out]
                n2018 = call-poly <vilib>:"Mean.vi"("X"=w4408) -> ("mean"=w4401:dbl)  [unwired: 1 out]
                n2019 = Subtract(x=w4402, y=w4401) -> (x-y=w4392:dbl)
                "Delta Fl. 2" <- w4392
                n2020 = Subtract(x=w4427, y=w4426) -> (x-y=w4424:dbl)
                "Delta Fl. 1" <- w4424
                n2021 = Initialize Array(w4424, 1 ("dimension size")) -> (w4421:dbl[])
                n2022 = Initialize Array(w4392, 1 ("dimension size")) -> (w4398:dbl[])
                n2023 = feedback #29(w4421) -> (w4422:dbl[])
                n2024 = Build Array (concatenate)(w4422, w4421) -> (w4420:dbl[])
                n2025 = feedback #30(w4398) -> (w4399:dbl[])
                n2026 = Build Array (concatenate)(w4399, w4398) -> (w4397:dbl[])
                n2027 = Select(t=w4421, s=w4393, f=w4420) -> (s? t:f=w4396:dbl[])
                n2028 = feedback-in #29(w4396) -> ()
                n2029 = Select(t=w4398, s=w4393, f=w4397) -> (s? t:f=w4395:dbl[])
                n2030 = feedback-in #30(w4395) -> ()
                n2031 = Build Array(w4396, w4395) -> (→"Save APD Deriv":dbl[][])
              }
            }
            "Progress" <- w4369
            "Progress 2" <- w4369
          }
        }
      }
    }
    n2032 = Bundle By Name(cluster=w2116, "Green FB Ch 0"=w2115, "Green FB Ch 1"=w2114) -> (w2094:T51)
    "Green FB Signals (V)" <- w2094
    n2033 = Unbundle By Name(w2094) -> ("Green FB Ch 2"=→"Green FB Plot":dbl)
    n2034 = local read "wait to reset values"() -> (w2186:bool)
    n2035 = Not(x=w2183) -> (.not. x?=w2187:bool)
    n2036 = And(x=w2187, y=w2186) -> (x .and. y?=w2188:bool)
    n2037 = case "Part of MCL raster scanning: returns to initial positions after scan done" shown="True" w2188 {
      tunnel: w2191 -> [w3459 w3466]
      tunnel: [w3459 w3465] -> w2190
      tunnel: w2185 -> [w3458 w3464]
      tunnel: [w3458 w3463] -> w2184
      frame False {
      }
      frame True {
        w3474 = 10.0 ("y")
        w3473 = 32767.0 ("y")
        # "to return scan values\nafter a synchronous \nAOM scan"
        n2038 = local read "AO2"() -> (w3467:dbl)
        n2039 = local read "AO1"() -> (w3468:dbl)
        n2040 = local write "wait to reset values"(FALSE ("wait to reset values")) -> ()
        n2041 = Multiply(x=w3468, y=w3473) -> (x*y=w3470:dbl)
        n2042 = Multiply(x=w3467, y=w3473) -> (x*y=w3472:dbl)
        n2043 = Divide(x=w3470, y=w3474) -> (x/y=w3469:dbl)
        n2044 = Divide(x=w3472, y=w3474) -> (x/y=w3471:dbl)
        n2045 = To Word Integer(number=w3469) -> (16bit integer=w3475:i16)
        n2046 = To Word Integer(number=w3471) -> (16bit integer=w3476:i16)
        n2047 = local read "Total Counts (ticks)"() -> (w3460:u32)
        n2048 = xnode "Read/Write Control"("FPGA VI Reference In"=w3466, "error in"=w3464, "AO1"=w3475, "AO2"=w3476, "MCL count"=w3460) -> ("FPGA VI Reference Out"=w3465:T19, "error out"=w3463:errorcluster)
